vi "Read Measurement (N Cycle Jitter).vi"(0 "VISA resource name":refnum<visa-resource-name>, 1 "Number Cycle (5)":i32 format="%.0g", 2 "Start Cycle (1)":i32 format="%.0g", 5 "Channel (1: Channel 1)":u16(ring) items=["Channel 1", "Channel 2", "Channel 3", "Channel 4", "Function 1", "Function 2", "Function 3", "Function 4", "Memory 1", "Memory 2", "Memory 3", "Memory 4"], 7 "Edge (0: Rising)":i32(ring) items=["Rising", "Falling"], 9 "Maximum Time (10000ms)":u32, 11 "error in (no error)":errorcluster) -> (4 "VISA resource name out":refnum<visa-resource-name>, 6 "N cycle jitter (s)":dbl, 15 "error out":errorcluster)   [LabVIEW 2009, in "Agilent 8000 Series.lvlib"]
doc: "Measures the N cycle jitter of the waveform. \n\nThis VI initiates an acquisition on the channel that the end-user defines. It then waits for the acquisition to complete, obtains a waveform measurement on the channel the end-user specifies, and returns the measurement value."
uses:
  Agilent 8000 Series.lvlib
  Low Level/Fetch Measurement (N Cycle Jitter).vi
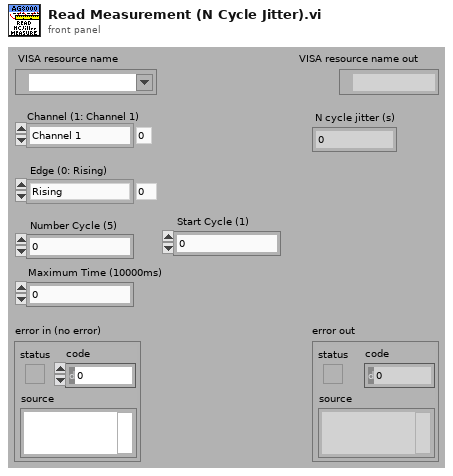
[diagram p1: front panel]
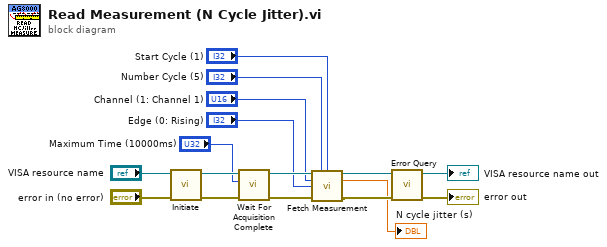
[diagram p0: block diagram]
diagram:
  n1 = call "Initiate.vi"("error in (no error)"="error in (no error)", "VISA resource name"="VISA resource name") -> ("error out"=w14:errorcluster, "VISA resource name out"=w13:refnum<visa-resource-name>)  [unwired: 8 in]
  n2 = call "Wait For Acquisition Complete.vi"("error in (no error)"=w14, "Maximum Time (10000ms)"="Maximum Time (10000ms)", "VISA resource name"=w13) -> ("error out"=w11:errorcluster, "VISA resource name out"=w12:refnum<visa-resource-name>)  [unwired: 7 in]
  n3 = call-poly "Fetch Measurement.vi"("VISA resource name"=w12, "Number Cycle (5)"="Number Cycle (5)", "Start Cycle (1)"="Start Cycle (1)", "Channel (1: Channel 1)"="Channel (1: Channel 1)", "Edge (0: Rising)"="Edge (0: Rising)", "error in (no error)"=w11) -> ("VISA resource name out"=w10:refnum<visa-resource-name>, "N cycle jitter (s)"=→"N cycle jitter (s)":dbl, "error out"=w9:errorcluster)  [unwired: 7 in]
  n4 = call "Error Query.vi"("error in (no error)"=w9, "VISA resource name"=w10) -> ("error out"=→"error out":errorcluster, "VISA resource name out"=→"VISA resource name out":refnum<visa-resource-name>)  [unwired: 6 in, 2 out]
